vi "Export Addon Configuration.vi"(8 "error in":errorcluster, 10 "export file path":path, 11 "FPGA addon refnum in":T1 format="%.0x") -> (0 "error out":errorcluster, 3 "FPGA addon refnum out":T1 format="%.0x")   [LabVIEW 2018, in "Scripting API.lvlib"]
uses:
  Scripting API.lvlib
  <vilib>/NI Veristand/Custom Device API/Custom Device Item Ref.ctl
  <vilib>/NI/NI VeriStand Custom Device Import and Export Tool/File Interface Class/File Interface.lvclass
  <vilib>/NI/NI VeriStand Custom Device Import and Export Tool/ImportExport.lvlib
  <vilib>/NI Veristand/Custom Device API/Custom Device API.lvlib
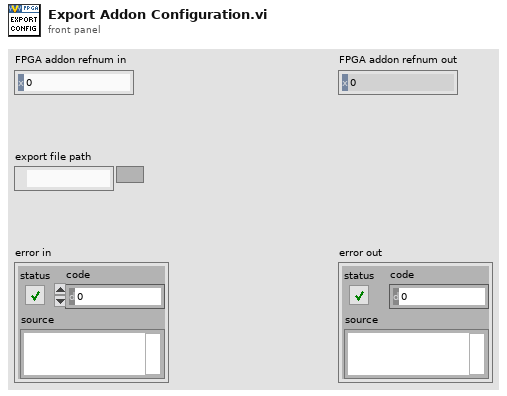
[diagram p1: front panel]
types:
  T1 = typedef "Custom Device API.lvlib/Custom Device Item Ref.ctl" = u64
  T2 = enum16{"open", "replace", "create", "open or create", "replace or create", "replace or create with confirmation"}
  T3 = typedef "Advanced System Definition.lvlib/SysDef.Export.ctl" = cluster{"Version":string, "Tree":T4[]}
  T4 = typedef "Advanced System Definition.lvlib/TreeItem.ctl" = cluster{"Item Info":T5, "Parent Path":string[], "Properties":T10[]}
  T5 = typedef "Advanced System Definition.lvlib/TreeItem.Info.ctl" = cluster{"Name":string, "Description":string, "GUID":string, "Is Channel":bool, "Channel":T6, "Is Waveform":bool, "Waveform":T8}
  T6 = typedef "Custom Device API.lvlib/Custom Device Channel.ctl" = cluster{"Type":T7, "Units":string, "Default Value":dbl, "Faultable":bool, "Scalable":bool}
  T7 = typedef "Custom Device API.lvlib/Custom Device Channel Type.ctl" = enum16{"Input", "Output"}
  T8 = typedef "Custom Device API.lvlib/Custom Device Waveform.ctl" = cluster{"Data Type":T9, "Units":string}
  T9 = typedef "Custom Device API.lvlib/Custom Device Waveform DataType.ctl" = enum16{"Double", "Complex Double"}
  T10 = typedef "Advanced System Definition.lvlib/TreeItem.Property.ctl" = cluster{"Name":string, "Type":i32, "Value":variant}
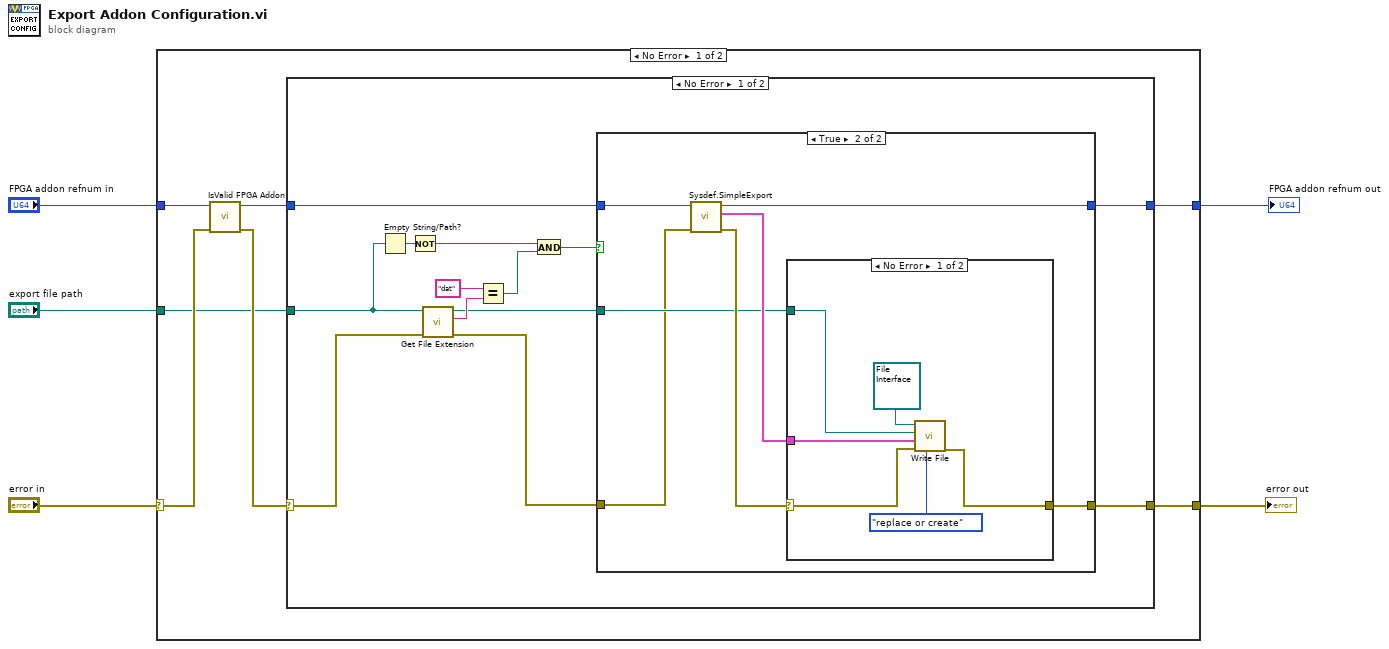
[diagram p0: block diagram]
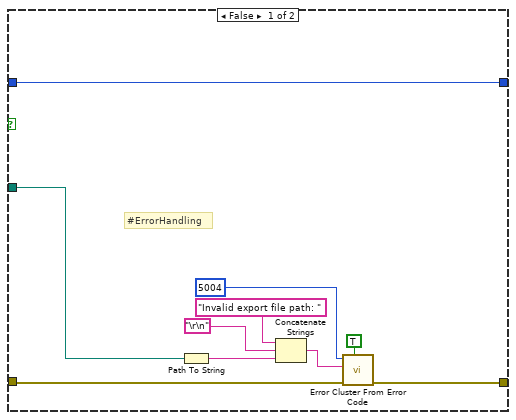
[diagram p2: hidden frame]
diagram:
  n1 = case shown="No Error" "error in" {
    selector: "error in" -> [w11 w52]
    tunnel: "FPGA addon refnum in" -> [w12 w53]
    tunnel: [w8 w53] -> w3
    tunnel: [w7 w52] -> w2
    tunnel: "export file path" -> [w6 _]
    frame No Error {
      n2 = call "IsValid FPGA Addon.vi"("error in"=w11, "FPGA Addon refnum in"=w12) -> ("error out"=w10:errorcluster, "FPGA Addon refnum out"=w9:T1)  [unwired: 8 in]
      n3 = case shown="No Error" w10 {
        selector: w10 -> [w21 w50]
        tunnel: w9 -> [w22 w51]
        tunnel: [w13 w51] -> w8
        tunnel: [w16 w50] -> w7
        tunnel: w6 -> [w20 _]
        frame No Error {
          n4 = Empty String/Path?(string/path=w20) -> (empty?=w23:bool)
          n5 = Not(x=w23) -> (.not. x?=w19:bool)
          n6 = call <vilib>:"Get File Extension.vi"("error in (no error)"=w21, "file"=w20) -> ("error out"=w17:errorcluster, "lowercase file extension"=w24:string, "dup file"=w15:path)  [unwired: 5 in, 2 out]
          n7 = Equal?(x="dat", y=w24) -> (x = y?=w18:bool)
          n8 = And(x=w19, y=w18) -> (x .and. y?=w14:bool)
          n9 = case shown="True" w14 {
            tunnel: w22 -> [w26 w40]
            tunnel: w17 -> [w29 w37]
            tunnel: [w28 w36] -> w16
            tunnel: w15 -> [w27 w38]
            tunnel: [w26 w39] -> w13
            frame False {
              # "#ErrorHandling"
              n10 = Path To String(path=w27) -> (string=w35:string)
              n11 = Concatenate Strings("Invalid export file path: " ("error message (\"\")"), "\r\n", w35) -> (w34:string)
              n12 = call <vilib>:"Error Cluster From Error Code.vi"("show call chain? (False)"=TRUE, "error in (no error)"=w29, "error message (\"\")"=w34, "error code (0)"=5004) -> ("error out"=w28:errorcluster)  [unwired: 5 in]
            }
            frame True {
              n13 = call <vilib>:"Sysdef.SimpleExport.vi"("error in (no error)"=w37, "ID"=w40) -> ("error out"=w42:errorcluster, "Export"=w41:T3, "ID out"=w39:u64)  [unwired: 7 in]
              n14 = case shown="No Error" w42 {
                selector: w42 -> [w46 w49]
                tunnel: [w47 w49] -> w36
                tunnel: w41 -> [w48 _]
                tunnel: w38 -> [w45 _]
                frame No Error {
                  n15 = call-dynamic "Write File.vi"("operation"=T2."replace or create", "error in (no error)"=w46, "Data"=w48, "datalog path (use dialog)"=w45, "File Interface in"=refnum<class "File Interface.lvclass"> refnum) -> ("error out"=w47:errorcluster)  [unwired: 6 in]
                }
                frame Error {
                }
              }
            }
          }
        }
        frame Error {
        }
      }
    }
    frame Error {
    }
  }
  "error out" <- w2
  "FPGA addon refnum out" <- w3
